vi "Read Measurement Data.vi"   [LabVIEW 2020, in "Yokogawa GX Series.lvlib"]
doc: "This VI select the type of read measurement data."
uses:
  <instrlib>/Yokogawa GX Series/Yokogawa GX Series.lvlib
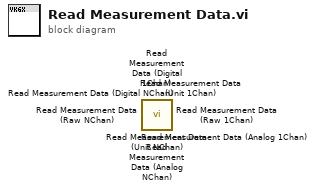
[diagram p0: block diagram]
diagram:
  n1 = call <instrlib>:"Read Measurement Data (Unit NChan).vi"() -> ()  [unwired: 10 in, 6 out]
  n2 = call <instrlib>:"Read Measurement Data (Unit 1Chan).vi"() -> ()  [unwired: 10 in, 6 out]
  n3 = call <instrlib>:"Read Measurement Data (Raw NChan).vi"() -> ()  [unwired: 8 in, 8 out]
  n4 = call <instrlib>:"Read Measurement Data (Raw 1Chan).vi"() -> ()  [unwired: 8 in, 8 out]
  n5 = call <instrlib>:"Read Measurement Data (Digital NChan).vi"() -> ()  [unwired: 9 in, 7 out]
  n6 = call <instrlib>:"Read Measurement Data (Digital 1Chan).vi"() -> ()  [unwired: 9 in, 7 out]
  n7 = call <instrlib>:"Read Measurement Data (Analog NChan).vi"() -> ()  [unwired: 8 in, 8 out]
  n8 = call <instrlib>:"Read Measurement Data (Analog 1Chan).vi"() -> ()  [unwired: 8 in, 8 out]
